vi "Hart_command_0.vi"(0 "VISA resource name":refnum<visa-resource-name>, 1 "retries":i32=5, 5 "milliseconds to wait":u32=1000, 7 "Short address":i32, 9 "search":bool, 11 "error in (no error)":errorcluster) -> (3 "output":u8[](array[numeric]) format="%02x", 4 "found header":bool, 6 "unique idenifier":u64 format="%x", 10 "long address":u64 format="%x", 12 "Address (array)":u8[](array[numeric]) format="%.0x", 14 "return count":u32, 15 "error out":errorcluster)   [LabVIEW 2016]
panel:
  out "short address out":i32
  out "dev ident code.":u32 format="%x"
  out "Dev. type":u8 format="%x"
  out "Man ID":u8 format="%x"
  out "Header\nindex":i32
  # "3"
  # "5"
  # "6"
  # "7"
  # "8"
  # "0"
  # "1"
  # "9"
  # "10"
  # "4"
  # "11"
  # "12"
  # "13"
  # "14"
  # "15"
  # "16"
  # "2"
  # "preamble"
  # "start delimiter"
  # "address"
  # "command"
  # "#data bytes"
  # "slave health"
  # "checksum"
  # "Man. Ident code"
  # "Dev. type"
  # "device ident. no."
  # "+"
  # "+"
  # "="
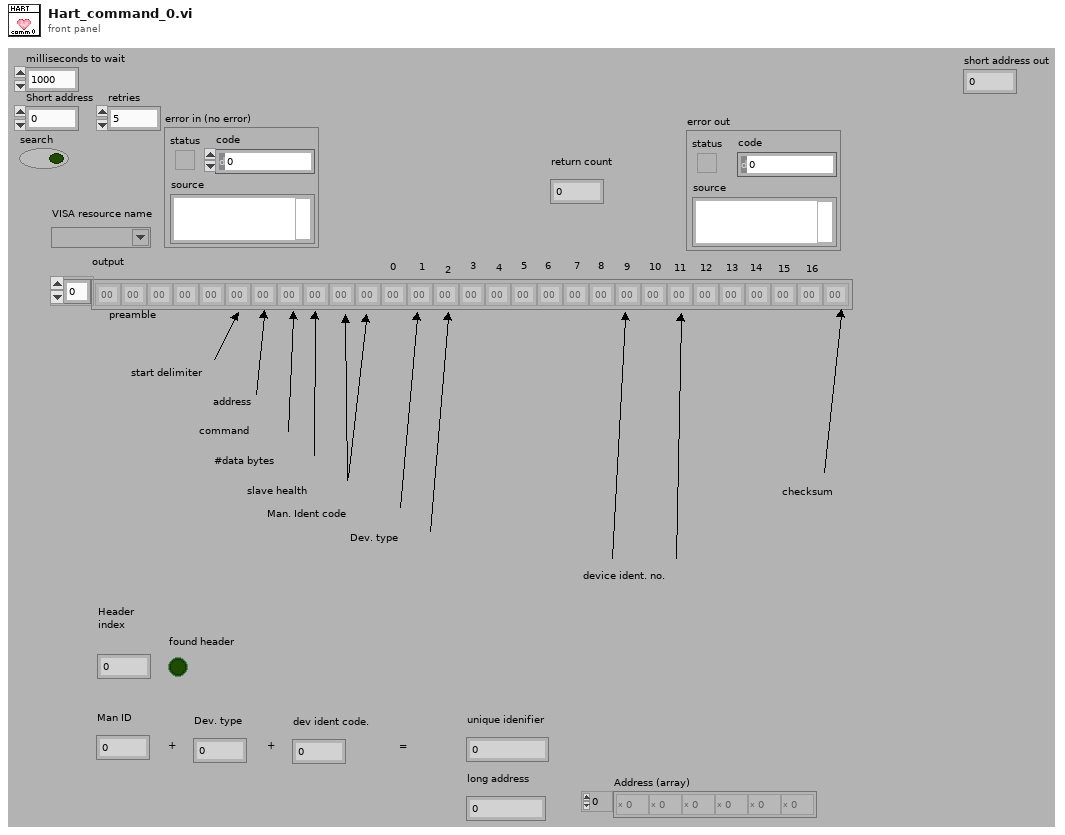
[diagram p1: front panel]
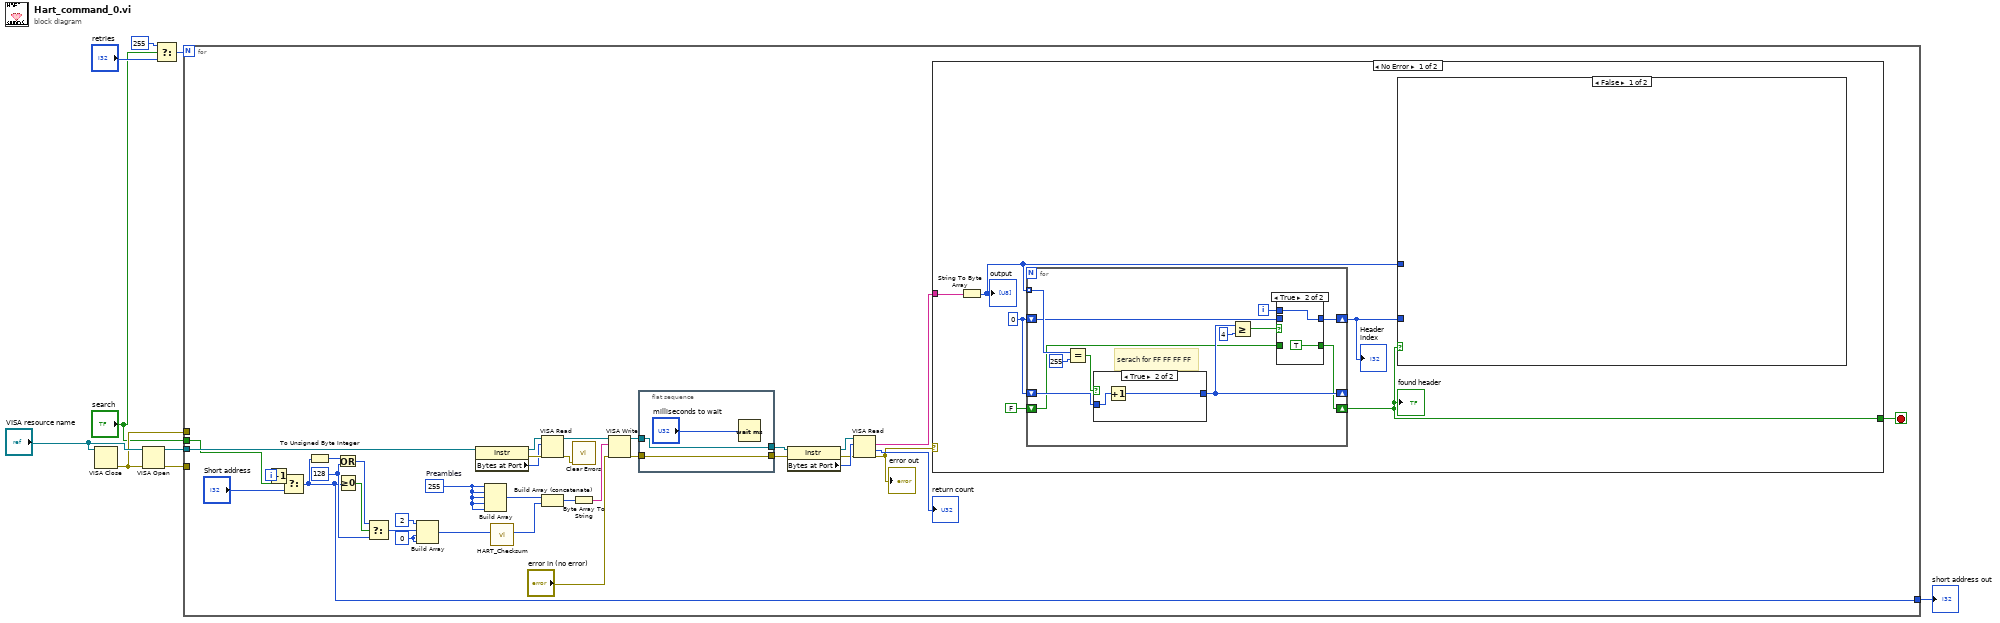
[diagram p0: block diagram]
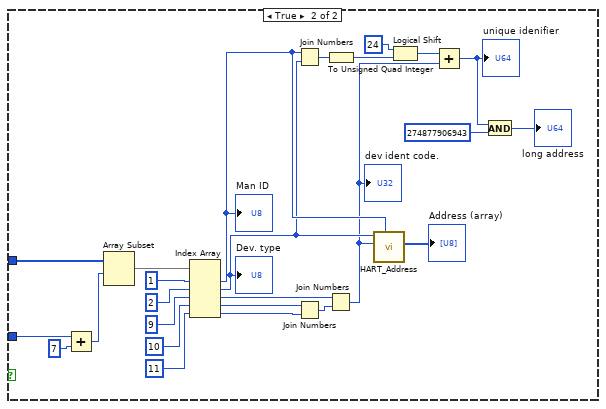
[diagram p2: hidden frame]
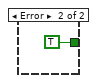
[diagram p5: hidden frame]
diagram:
  n1 = VISA Close(VISA resource name="VISA resource name") -> (error out=w6:errorcluster)  [unwired: 1 in]
  n2 = VISA Open(error in (no error)=w6, VISA resource name="VISA resource name") -> (VISA resource name=w8:refnum<visa-resource-name>, error out=w7:errorcluster)  [unwired: 3 in]
  n3 = Select(t=255, s="search", f="retries") -> (s? t:f=w5:i32)
  n4 = for {
    N: w5 -> [_]
    tunnel: w8 -> [w16]
    tunnel: w6 -> [_]
    tunnel: w7 -> [_]
    tunnel: [w11] -> w2
    tunnel: "search" -> [w13]
    i -> [w12]
    stop <- w15 stop-if-true
    w32 = u8 255  # Preambles
    w20 = u8 0
    w38 = u8 128
    n5 = Increment(x=w12) -> (x+1=w10:i32)
    n6 = Select(t=w10, s=w13, f="Short address") -> (s? t:f=w11:i32)
    n7 = To Unsigned Byte Integer(number=w11) -> (unsigned 8bit integer=w37:u8)
    n8 = Or(x=w37, y=w38) -> (x .or. y?=w39:u8)
    n9 = Greater Or Equal To 0?(x=w11) -> (x >= 0?=w31:bool)
    n10 = Select(t=w39, s=w31, f=w38) -> (s? t:f=w40:u8)
    n11 = Build Array(u8 2, w40, w20, w20) -> (w33:u8[])
    n12 = property class="Instr"(reference=w16) -> (reference out=w42:refnum<visa-resource-name>, error out=w43:errorcluster, "Bytes at Port"=w41:u32)  [unwired: 1 in]
    n13 = Build Array(w32, w32, w32, w32, w32) -> (w34:u8[])
    n14 = call "HART_Checksum.vi"("message"=w33) -> ("message + chk"=w35:u8[])  [unwired: 9 in, 1 out]
    n15 = VISA Read(VISA resource name=w42, byte count=w41, error in (no error)=w43) -> (VISA resource name out=w45:refnum<visa-resource-name>, error out=w44:errorcluster)  [unwired: 2 out]
    n16 = Build Array (concatenate)(w34, w35) -> (w36:u8[])
    n17 = call <vilib>:"Clear Errors.vi"("error in (no error)"=w44) -> ()  [unwired: 5 in, 2 out]
    n18 = Byte Array To String(unsigned byte array=w36) -> (string=w21:string)
    n19 = VISA Write(VISA resource name=w45, write buffer=w21, error in (no error)="error in (no error)") -> (VISA resource name out=w23:refnum<visa-resource-name>, error out=w24:errorcluster)  [unwired: 1 out]
    n20 = flat-sequence {
      tunnel: w23 -> [w48]
      tunnel: w24 -> [w47]
      tunnel: [w48] -> w27
      tunnel: [w47] -> w25
      frame #0 {
        n21 = Wait (ms)(milliseconds to wait="milliseconds to wait") -> ()  [unwired: 1 out]
      }
    }
    n22 = property class="Instr"(reference=w27, error in=w25) -> (reference out=w28:refnum<visa-resource-name>, error out=w26:errorcluster, "Bytes at Port"=w29:u32)
    n23 = VISA Read(VISA resource name=w28, byte count=w29, error in (no error)=w26) -> (read buffer=w18:string, return count=→"return count":u32, error out=w17:errorcluster)  [unwired: 1 out]
    "error out" <- w17
    n24 = case shown="No Error" w17 {
      tunnel: w18 -> [w54 _]
      tunnel: [w49 TRUE] -> w15
      frame No Error {
        w53 = 0
        n25 = String To Byte Array(string=w54) -> (unsigned byte array=w51:u8[])
        "output" <- w51
        n26 = for {
          tunnel: w51 -> [w91] mode=indexing
          shift-right: [w87] -> _
          shift-left: w53 -> [w90]
          shift-right: [w84] -> w50
          shift-left: w53 -> [w86]
          shift-right: [w81] -> w49
          shift-left: FALSE -> [w80]
          i -> [w85]
          # "serach for FF FF FF FF"
          n27 = Equal?(x=w91, y=u8 255 ("element")) -> (x = y?=w83:bool)
          n28 = case shown="True" w83 {
            tunnel: w90 -> [_ w97]
            tunnel: [_ w96] -> w87
            frame False {
            }
            frame True {
              n29 = Increment(x=w97) -> (x+1=w96:i32)
            }
          }
          n30 = Greater Or Equal?(x=w87, y=4) -> (x >= y?=w82:bool)
          n31 = case shown="True" w82 {
            tunnel: w86 -> [w93 _]
            tunnel: w85 -> [_ w95]
            tunnel: [w93 w95] -> w84
            tunnel: [w92 TRUE] -> w81
            tunnel: w80 -> [w92 _]
            frame False {
            }
            frame True {
            }
          }
        }
        "found header" <- w49
        "Header\nindex" <- w50
        n32 = case shown="False" w49 {
          tunnel: w51 -> [_ w79]
          tunnel: w50 -> [_ w77]
          frame False {
          }
          frame True {
            n33 = Add(x=w77, y=7) -> (x+y=w78:i32)
            n34 = Array Subset(array=w79, index=w78) -> (w75:u8[])  [unwired: 1 in]
            n35 = Index Array(array=w75, index #1=1 ("index"), index #2=2 ("index"), index #3=9 ("index"), index #4=10 ("index"), index #5=11 ("index")) -> (element #1=w58:u8, element #2=w57:u8, element #3=w69:u8, element #4=w72:u8, element #5=w71:u8)
            "Man ID" <- w58
            "Dev. type" <- w57
            n36 = Join Numbers(hi=w58, lo=w57) -> ((hi.lo)=w64:u16)
            n37 = Join Numbers(hi=w72, lo=w71) -> ((hi.lo)=w70:u16)
            n38 = To Unsigned Quad Integer(1:w64) -> (0:w63:u64)
            n39 = Join Numbers(hi=w69, lo=w70) -> ((hi.lo)=w56:u32)
            "dev ident code." <- w56
            n40 = call "HART_Address.vi"("Primary Master"=w58, "Tag no. (device ID)"=w56, "Dev Type"=w57) -> ("Address"=→"Address (array)":u8[])  [unwired: 8 in]
            n41 = Logical Shift(y=i8 24, x=w63) -> (x << y=w62:u64)
            n42 = Add(x=w62, y=w56) -> (x+y=w61:u64)
            "unique idenifier" <- w61
            n43 = And(x=w61, y=u64 274877906943) -> (x .and. y?=→"long address":u64)
          }
        }
      }
      frame Error {
      }
    }
  }
  "short address out" <- w2
